vi "N5224B_Initialize(SubVI).vi"(11 "Cluster in":T1={"Power Level"=-5.0, "Center Freq"=18000000000.0, "Span Freq"=2000000000.0, "Sweep Points"=5, "IF Bandwidth"=500.0, "Average Count"=5, "error"={"status"=FALSE, "code"=0, "source"=""}, "Instrument"="GPIB0::10::INSTR", "Mode"=0, "Motor Range"=90, "Motor Step"=10, "VISA"=""} {"Motor Step" items=["1 deg"=1, "3 deg"=3, "5 deg"=5, "10 deg"=10]; "Motor Range" items=["360 deg"=360, "180 deg"=180, "90 deg"=90]; "Mode" items=["Create", "Delete", "Select"]; "IF Bandwidth" format="%.3p"; "Span Freq" format="%.3p"; "Center Freq" format="%.3p"; "Power Level" format="%.2p"}) -> (3 "Cluster out":T1={"Power Level"=-5.0, "Center Freq"=18000000000.0, "Span Freq"=2000000000.0, "Sweep Points"=5, "IF Bandwidth"=500.0, "Average Count"=5, "error"={"status"=FALSE, "code"=0, "source"=""}, "Instrument"="GPIB0::10::INSTR", "Mode"=0, "Motor Range"=90, "Motor Step"=10, "VISA"=""} {"Motor Step" items=["1 deg"=1, "3 deg"=3, "5 deg"=5, "10 deg"=10]; "Motor Range" items=["360 deg"=360, "180 deg"=180, "90 deg"=90]; "Mode" items=["Create", "Delete", "Select"]; "IF Bandwidth" format="%.3p"; "Span Freq" format="%.3p"; "Center Freq" format="%.3p"; "Power Level" format="%.2p"})   [LabVIEW 2020]
uses:
  Chamber_2018/ControlCluster.ctl
  <instrlib>/Agilent PNA Series/Agilent PNA Series.lvlib
panel:
  # "Hz"
  # "Hz"
  # "Hz"
  # "dBm"
  # "Hz"
  # "Hz"
  # "Hz"
  # "dBm"
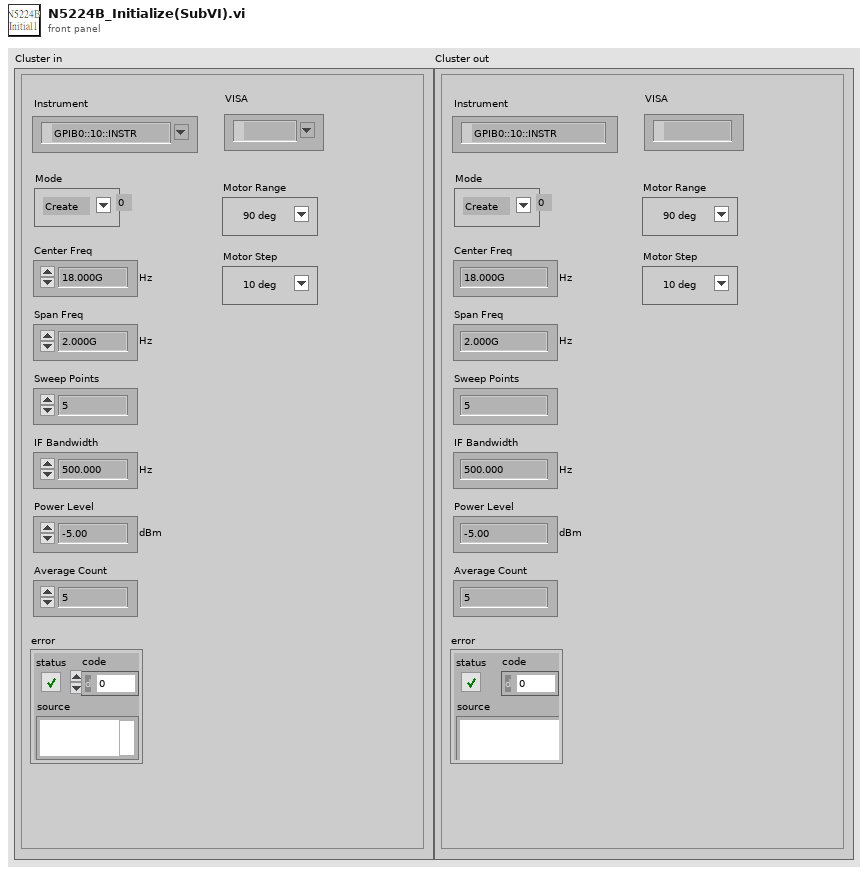
[diagram p1: front panel]
types:
  T1 = typedef "ControlCluster.ctl" = cluster{"Power Level":dbl, "Center Freq":dbl, "Span Freq":dbl, "Sweep Points":u32, "IF Bandwidth":dbl, "Average Count":i32, "error":errorcluster, "Instrument":refnum<visa-resource-name>, "Mode":u16, "Motor Range":u16, "Motor Step":u16, "VISA":refnum<visa-resource-name>}
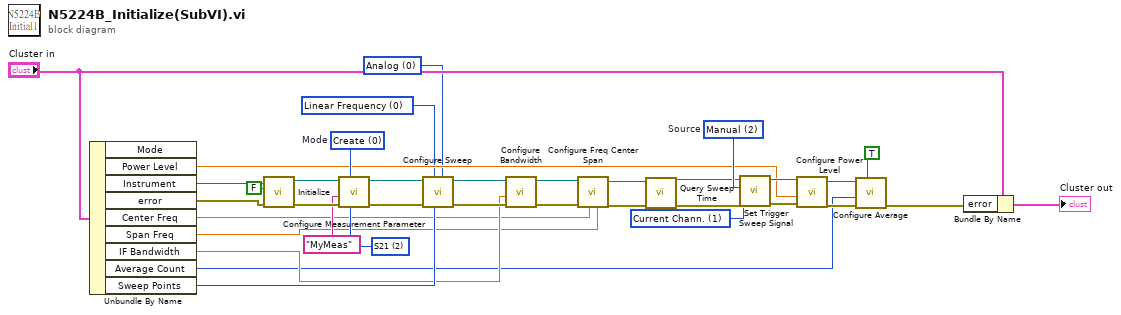
[diagram p0: block diagram]
diagram:
  w1 = u16 1 items=["All Channels", "Current Chann."] ("Trigger Scope (0: All Channels )")
  w8 = 0 items=["Analog", "Stepped"] ("Sweep Gen Type (0: Analog)")
  w9 = 0 items=["Linear Frequency", "Log Frequency", "Power Sweep", "CW Time"] ("Sweep Type (0: Linear Frequency)")
  w20 = 2 items=["S11", "S12", "S21", "S22", "A", "B", "R1", "R2", "A/B", "B/A"] ("Measurement Type (0: S11)")
  w24 = u16 2 items=["Immediate", "External", "Manual"]  # Source
  w34 = u16 0 items=["Create", "Delete", "Select"]  # Mode
  n1 = Unbundle By Name("Cluster in") -> ("Power Level"=w13:dbl, "Instrument"=w23:refnum<visa-resource-name>, "error"=w21:errorcluster, "Center Freq"=w17:dbl, "Span Freq"=w16:dbl, "IF Bandwidth"=w18:dbl, "Average Count"=w10:i32, "Sweep Points"=w19:u32)  [unwired: 1 out]
  n2 = call <instrlib>:"Initialize.vi"("error in (no error)"=w21, "ID Query (T: Check)"=FALSE, "Instrument Resource Name"=w23) -> ("error out"=w27:errorcluster, "dup VISA session"=w26:refnum<visa-resource-name>)  [unwired: 7 in]
  n3 = call <instrlib>:"Configure Measurement Parameter.vi"("Measurement Type (0: S11)"=w20, "Mode (0: Create)"=w34, "Error In (no error)"=w27, "Measurement Name (MY_MEAS)"="MyMeas", "VISA Resource Name"=w26) -> ("Error Out"=w29:errorcluster, "VISA Resource Name Out"=w28:refnum<visa-resource-name>)  [unwired: 5 in]
  n4 = call <instrlib>:"Configure Sweep.vi"("Sweep Gen Type (0: Analog)"=w8, "Sweep Points (201)"=w19, "Sweep Type (0: Linear Frequency)"=w9, "Error In (no error)"=w29, "VISA session"=w28) -> ("Error Out"=w30:errorcluster, "dup VISA session"=w31:refnum<visa-resource-name>)  [unwired: 5 in]
  n5 = call <instrlib>:"Configure Bandwidth.vi"("Error In (no error)"=w30, "Bandwidth (20.0E+3)"=w18, "VISA session"=w31) -> ("Error Out"=w33:errorcluster, "dup VISA session"=w32:refnum<visa-resource-name>)  [unwired: 7 in]
  n6 = call <instrlib>:"Configure Freq Center Span.vi"("Span Freq (2.9997 E+9)"=w16, "Center Freq (1.50015 E+9)"=w17, "Error In (no error)"=w33, "VISA session"=w32) -> ("Error Out"=w4:errorcluster, "dup VISA session"=w5:refnum<visa-resource-name>)  [unwired: 6 in]
  n7 = call <instrlib>:"Query Sweep Time.vi"("Error In (no error)"=w4, "VISA Resource Name"=w5) -> ("Error Out"=w3:errorcluster, "VISA Resource Name Out"=w2:refnum<visa-resource-name>)  [unwired: 7 in, 1 out]
  n8 = call <instrlib>:"Set Trigger Sweep Signal.vi"("Error In (no error)"=w3, "Trigger Scope (0: All Channels )"=w1, "Source (0: Immediate)"=w24, "VISA session"=w2) -> ("Error Out"=w15:errorcluster, "dup VISA session"=w14:refnum<visa-resource-name>)  [unwired: 6 in]
  n9 = call <instrlib>:"Configure Power Level.vi"("Error In (no error)"=w15, "Power Level (0.0)"=w13, "VISA Resource Name"=w14) -> ("Error Out"=w12:errorcluster, "VISA Resource Name Out"=w11:refnum<visa-resource-name>)  [unwired: 7 in]
  n10 = call <instrlib>:"Configure Average.vi"("Average State (F: Off)"=TRUE, "Error In (no error)"=w12, "Average Count (1)"=w10, "VISA Resource Name"=w11) -> ("Error Out"=w7:errorcluster)  [unwired: 6 in, 1 out]
  n11 = Bundle By Name(cluster="Cluster in", "error"=w7) -> (→"Cluster out":T1)
